vi "Check Step Order.vi"(8 "error in (no error)":refnum<class "MultiErrors.lvclass">, 11 "Sequence Validation in":refnum<class "Sequence Validation.lvclass">) -> (0 "error out":refnum<class "MultiErrors.lvclass">, 3 "Sequence Validation out":refnum<class "Sequence Validation.lvclass">)   [LabVIEW 2020, in "VolatusSeq.lvlib" / "Sequence Validation.lvclass"]
uses:
  Sequence Validation.lvclass
  Sequence Validation.lvclass/Sequence Validation.ctl
  Sequence Config/Sequence Config.lvclass
  VolatusErrorUtilities/MultiErrors/MultiErrors.lvclass
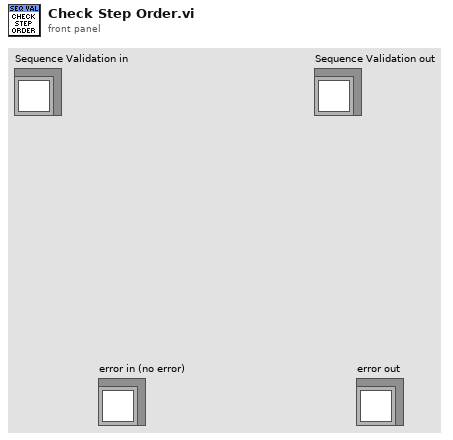
[diagram p1: front panel]
types:
  T1 = typedef "VolatusSeqConfig.lvlib/State.ctl" = cluster{"Name":string, "Steps":T2[], "Transitions":refnum<class "Transition Config.lvclass">[], "Comment":string, "Color":string, "Seq Name":string, "Report Conditions":bool}
  T2 = typedef "VolatusSeqConfig.lvlib/Step.ctl" = cluster{"Time":dbl, "Commands":refnum<class "Command Config.lvclass">[]}
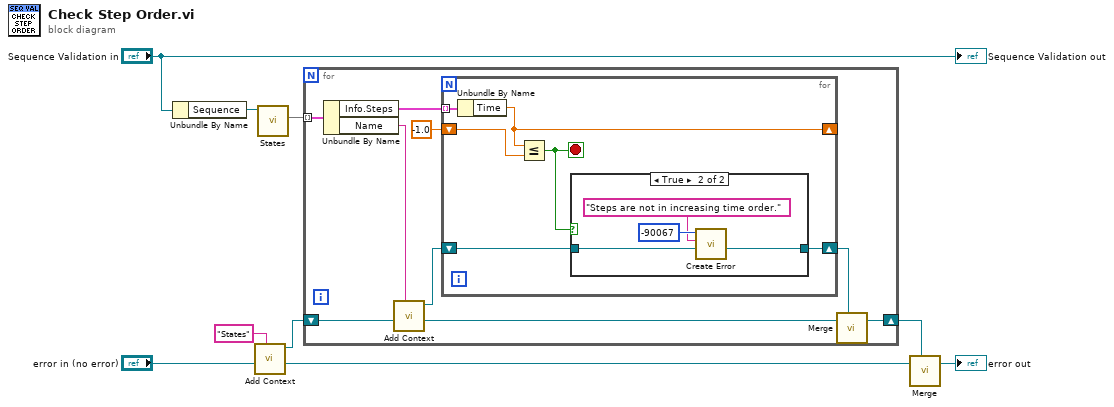
[diagram p0: block diagram]
diagram:
  n1 = Unbundle By Name("Sequence Validation in") -> ("Sequence"=w8:refnum<class "Sequence Config.lvclass">)
  n2 = call "Add Context.vi"("Context"="States", "MultiErrors in"="error in (no error)") -> ("Original Context"=w4:refnum<class "MultiErrors.lvclass">, "Added Context"=w3:refnum<class "MultiErrors.lvclass">)  [unwired: 8 in]
  n3 = call "States.vi"("Sequence Config in"=w8) -> ("States"=w7:map{string, T1})  [unwired: 8 in, 2 out]
  n4 = for {
    tunnel: w7 -> [w18] mode=indexing
    shift-right: [w10] -> w1
    shift-left: w3 -> [w17]
    n5 = Unbundle By Name(w18) -> ("Info.Steps"=w14:T2[], "Name"=w16:string)
    n6 = call "Add Context.vi"("Context"=w16, "MultiErrors in"=w17) -> ("Original Context"=w12:refnum<class "MultiErrors.lvclass">, "Added Context"=w15:refnum<class "MultiErrors.lvclass">)  [unwired: 8 in]
    n7 = for {
      tunnel: w14 -> [w24] mode=indexing
      shift-right: [w22] -> _
      shift-left: -1.0 -> [w23]
      shift-right: [w19] -> w11
      shift-left: w15 -> [w21]
      stop <- w20 stop-if-true
      n8 = Unbundle By Name(w24) -> ("Time"=w22:dbl)
      n9 = Less Or Equal?(x=w22, y=w23) -> (x <= y?=w20:bool)
      n10 = case shown="True" w20 {
        tunnel: w21 -> [w25 w29]
        tunnel: [w25 w26] -> w19
        frame False {
        }
        frame True {
          n11 = call "Create Error.vi"("MultiErrors in"=w29, "Message"="Steps are not in increasing time order.", "Code"=-90067) -> ("MultiErrors out"=w26:refnum<class "MultiErrors.lvclass">)  [unwired: 8 in]
        }
      }
    }
    n12 = call "Merge.vi"("First Error In"=w12, "Second Error In"=w11) -> ("MultiErrors out"=w10:refnum<class "MultiErrors.lvclass">)  [unwired: 5 in]
  }
  n13 = call "Merge.vi"("First Error In"=w4, "Second Error In"=w1) -> ("MultiErrors out"=→"error out":refnum<class "MultiErrors.lvclass">)  [unwired: 5 in]
  "Sequence Validation out" <- "Sequence Validation in"
